vi "__keysight_open_chopper.vi"() -> ()   [LabVIEW 2013]
panel:
  in  "Frequency Parameters":T1={"Coupling"=FALSE, "Frequency 2 (MHz)"=2.0, "Frequency 1 (MHz)"=3.0, "WAVEFORM"=enum."PULSE"} {"Frequency 1 (MHz)" min=0.0 max=14.5; "Frequency 2 (MHz)" min=0.0 max=14.5}
  in  "Keysight Connection":T2={"Type"=1, "VISA"="TCPIP0::192.168.0.8::inst0::INSTR", "GPIB"="10"} {"Type" items=["VISA", "GPIB"]}
  out "resulting string 2":string=":PULS:WIDTH1 2.000NS\n:PULS:WIDTH2 2.000NS\n:PULS:DEL1 0.000NS\n:PULS:DEL2 3.000NS\n"
  out "Keysight settings":T3 {"Frequency 1 (Hz)" format="%#_6p"; "Frequency 2 (Hz)" format="%#_6p"}
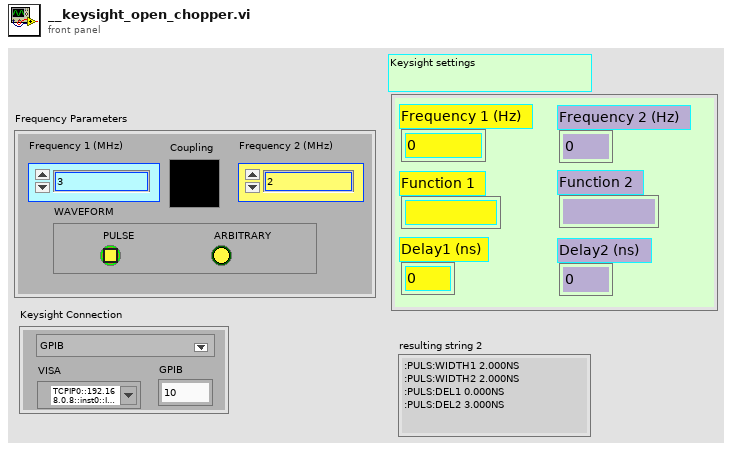
[diagram p1: front panel]
types:
  T1 = cluster{"Coupling":bool, "Frequency 2 (MHz)":dbl, "Frequency 1 (MHz)":dbl, "WAVEFORM":enum32{"PULSE", "ARBITRARY"}}
  T2 = cluster{"Type":u16, "VISA":refnum<visa-resource-name>, "GPIB":string}
  T3 = cluster{"Frequency 2 (Hz)":dbl, "Function 2":string, "Delay2 (ns) ":dbl, "Frequency 1 (Hz)":dbl, "Function 1":string, "Delay1 (ns)":dbl}
  T4 = cluster{"Ouput 1":bool, "Ouput 2":bool, "Ouput 1 Neg":bool, "Ouput 2 Neg":bool}
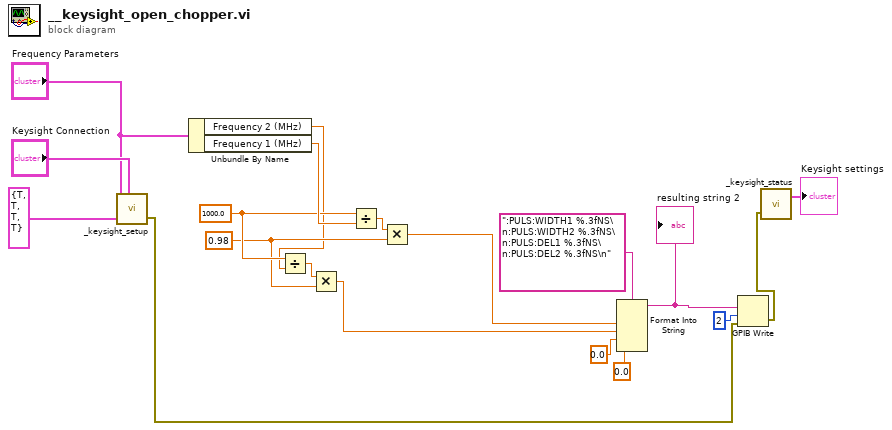
[diagram p0: block diagram]
diagram:
  w3 = 0.98 ("y")
  w4 = 1000.0 ("x")
  n1 = call "_keysight_setup.vi"("Frequency Parameters"="Frequency Parameters", "Outputs"=T4 {"Ouput 1"=TRUE, "Ouput 2"=TRUE, "Ouput 1 Neg"=TRUE, "Ouput 2 Neg"=TRUE}, "Keysight Connection"="Keysight Connection") -> ("error out"=w11:errorcluster)  [unwired: 3 in]
  n2 = Unbundle By Name("Frequency Parameters") -> ("Frequency 2 (MHz)"=w2:dbl, "Frequency 1 (MHz)"=w8:dbl)
  n3 = Divide(x=w4, y=w2) -> (x/y=w6:dbl)
  n4 = Multiply(x=w6, y=w3) -> (x*y=w5:dbl)
  n5 = Divide(x=w4, y=w8) -> (x/y=w7:dbl)
  n6 = Multiply(x=w7, y=w3) -> (x*y=w1:dbl)
  n7 = Format Into String(format string=":PULS:WIDTH1 %.3fNS\n:PULS:WIDTH2 %.3fNS\n:PULS:DEL1 %.3fNS\n:PULS:DEL2 %.3fNS\n", w1, w5, 0.0 ("Ch1 Delay"), 0.0 ("Ch2 Delay")) -> (resulting string=w14:string)  [unwired: 2 in, 1 out]
  "resulting string 2" <- w14
  n8 = GPIB Write(1:w14, 2:2, 3:w11) -> (6:w10:errorcluster)  [unwired: 2 in, 1 out]
  n9 = call "_keysight_status.vi"("error in"=w10) -> ("Keysight settings"=→"Keysight settings":T3)  [unwired: 2 in, 1 out]
